vi "Find Matching Controls.vi"(9 "Qualified Name Array":string[](array[string]), 11 "Ctl Data":T1[](array[typedef])) -> (3 "Ctl Data out":T1[](array[typedef]))   [LabVIEW 2020, in "MacroAssert.lvlib"]
doc: "Finds controls in <B>Ctl Data</B> whose qualified names match <B>Qualified Name Array</B>."
uses:
  MacroAssert.lvlib
  CTLs/Control Map Control Data.ctl
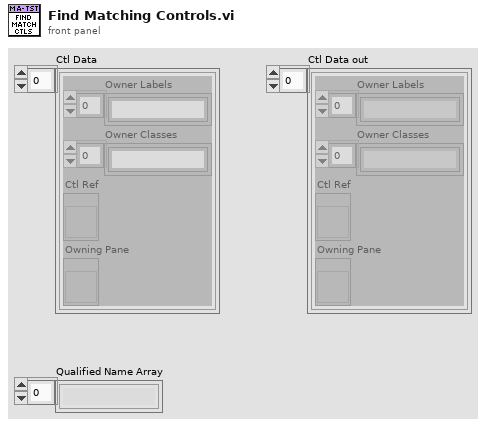
[diagram p1: front panel]
types:
  T1 = typedef "MacroAssert.lvlib/Control Map Control Data.ctl" = cluster{"Owner Labels":string[], "Owner Classes":string[], "Ctl Ref":refnum<vi>, "Owning Pane":refnum<vi>}
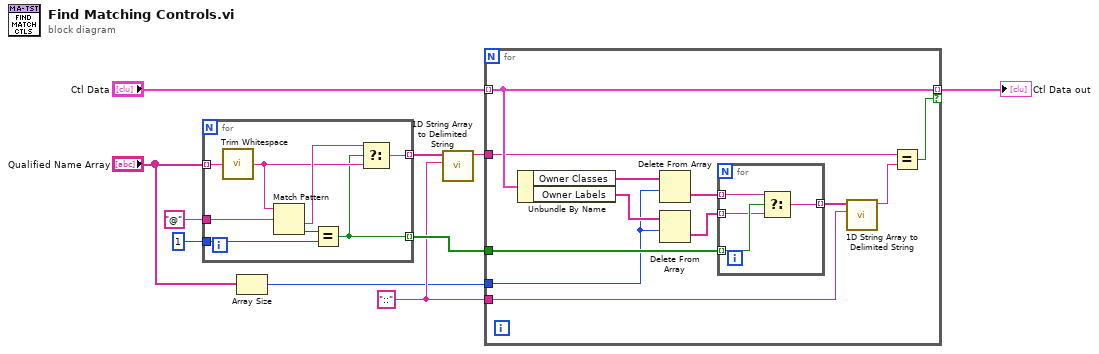
[diagram p0: block diagram]
diagram:
  w5 = "::" ("delimiter")
  n1 = for {
    tunnel: "Qualified Name Array" -> [w18] mode=indexing
    tunnel: [w15] -> w7 mode=indexing
    tunnel: [w11] -> w8 mode=indexing
    tunnel: "@" ("search string/char (-)") -> [w14]
    tunnel: 1 ("y") -> [w12]
    n2 = call-poly <vilib>:"Trim Whitespace.vi"("string"=w18) -> ("trimmed string"=w16:string)  [unwired: 1 in]
    n3 = Match Pattern(string=w16, regular expression=w14) -> (after substring=w17:string, offset past match=w13:i32)  [unwired: 1 in, 2 out]
    n4 = Equal?(x=w13, y=w12) -> (x = y?=w11:bool)
    n5 = Select(t=w17, s=w11, f=w16) -> (s? t:f=w15:string)
  }
  n6 = Array Size(array="Qualified Name Array") -> (size(s)=w1:i32)
  n7 = call-poly <vilib>:"1D String Array to Delimited String.vi"("delimiter"=w5, "string array"=w7) -> ("delimited string"=w6:string)  [unwired: 9 in]
  n8 = for {
    tunnel: "Ctl Data" -> [w29] mode=indexing
    tunnel: [w29] -> w9 mode=indexing if=w30
    tunnel: w8 -> [w27]
    tunnel: w6 -> [w28]
    tunnel: w5 -> [w26]
    tunnel: w1 -> [w19]
    n9 = Unbundle By Name(w29) -> ("Owner Classes"=w23:string[], "Owner Labels"=w21:string[])
    n10 = Delete From Array(array=w23, length=w19) -> (deleted portion=w22:string[])  [unwired: 1 in, 1 out]
    n11 = Delete From Array(array=w21, length=w19) -> (deleted portion=w20:string[])  [unwired: 1 in, 1 out]
    n12 = for {
      tunnel: w22 -> [w33] mode=indexing
      tunnel: w20 -> [w32] mode=indexing
      tunnel: w27 -> [w34] mode=indexing
      tunnel: [w31] -> w25 mode=indexing
      n13 = Select(t=w33, s=w34, f=w32) -> (s? t:f=w31:string)
    }
    n14 = call-poly <vilib>:"1D String Array to Delimited String.vi"("delimiter"=w26, "string array"=w25) -> ("delimited string"=w24:string)  [unwired: 9 in]
    n15 = Equal?(x=w28, y=w24) -> (x = y?=w30:bool)
  }
  "Ctl Data out" <- w9
